vi "S8300E_Ping_Port1_WIH.vi"() -> ()   [LabVIEW 2011]
panel:
  out "PRELOG2":string
  out "PRELOG1":string
  out "KEYWORD2_AfterLogin":string
  out "log1":string
  out "Debug View":string
  out "VISA resource name out":refnum<visa-resource-name>
  out "Log":string
  out "IP list":cluster{"PORT3 IP":string, string}[](array[cluster])
  out "Msg":string
  out "Error Code List":string[](array[string])
  out "PORT3 IP":string
  out "PORT2 IP":string
  out "PORT1IP":string
  out "BEGIN TIME":u32
  out "進行狀況":string
  # "Error Code:NETPORT1\nError Code:NETPORT2\nError Code:NETPORT3"
  # "S8300E Ping port1 IP (接UART COM9)"
  # "2015-6-1"
  # "Step1:PING UUT PORT1 IP\nStep2:PING UUT PORT2 IP\nStep3:PING UUT PORT3 IP"
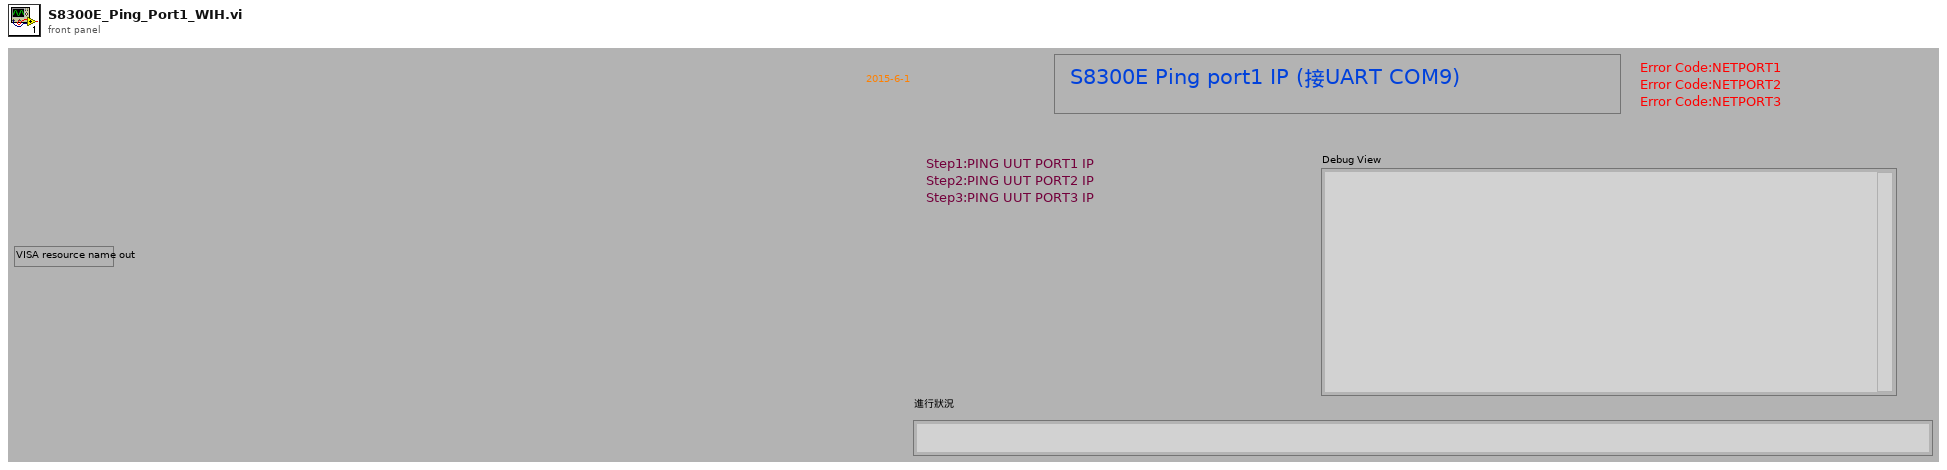
[diagram p1: front panel]
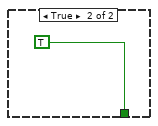
[diagram p6: hidden frame]
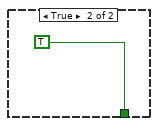
[diagram p9: hidden frame]
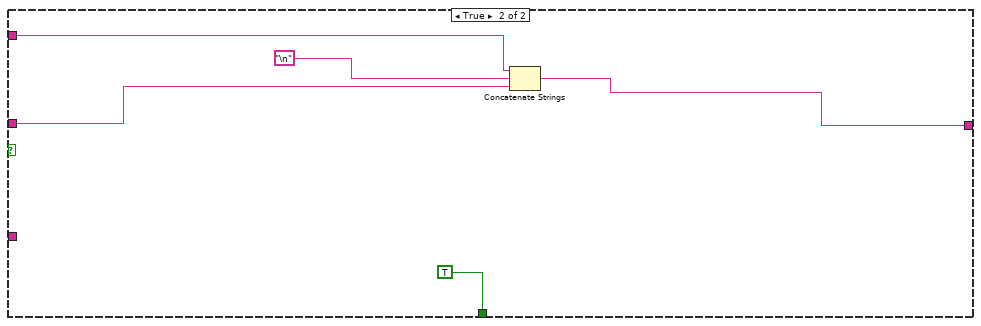
[diagram p11: hidden frame]
diagram:
  n1 = flat-sequence {
    tunnel: [w47] -> w3
    tunnel: [w46] -> w2
    tunnel: w3 -> [w53]
    tunnel: w2 -> [w52]
    tunnel: [w50] -> w1
    tunnel: w1 -> [w71]
    frame #0 {
      n2 = Tick Count (ms)() -> (millisecond timer value=→"BEGIN TIME":u32)
    }
    frame #1 {
      n3 = property on="進行狀況" class="Str"("Blinking"=TRUE) -> ()  [unwired: 2 in, 2 out]
      "進行狀況" <- "進入測試準備中...." ("進行狀況")
      "Debug View" <- ""
    }
    frame #2 {
      n4 = call "SUB_SearchFile_inFolder.vi"("Search Filename in Folder"="S8300E_sfcs_misc.txt") -> ("File Existing True/Flase"=w8:bool)  [unwired: 1 in]
      n5 = case shown="False" w8 {
        frame False {
          n6 = flat-sequence {
            frame #0 {
              n7 = call "Display Message to User"() -> ()  [unwired: 10 in, 2 out]
            }
            frame #1 {
              n8 = call "SUB_Writelog.vi"("Pass/Fail"="Fail:S8300E_Ping_Port1") -> ()  [unwired: 2 in]
            }
            frame #2 {
              n9 = Quit LabVIEW(quit? (T)=TRUE) -> ()
            }
          }
        }
        frame True {
        }
      }
    }
    frame #3 {
      w19 = "\r"
      n10 = call "SUB_ReadScript_File.vi"("Script FileName"="S8300E_sfcs_misc.txt" ("Search Filename in Folder")) -> ("text"=w16:string)  [unwired: 1 in, 2 out]
      n11 = call "SUB_FindSpecificString.vi"("Find this String"="TELNET_KEYWORD2_AFTERLOG_IN=", "String data"=w16) -> ("before \"; \" string"=→"KEYWORD2_AfterLogin":string, "Found"=w12:bool)  [unwired: 2 in]
      n12 = call "SUB_FindSpecificString.vi"("Find this String"="UUT_PORT2_IP=", "String data"=w16) -> ("before \"; \" string"=w22:string, "Found"=w26:bool)  [unwired: 2 in]
      "PORT2 IP" <- w22
      n13 = call "SUB_FindSpecificString.vi"("Find this String"="UUT_PORT3_IP=", "String data"=w16) -> ("before \"; \" string"=w21:string, "Found"=w24:bool)  [unwired: 2 in]
      "PORT3 IP" <- w21
      n14 = call "SUB_FindSpecificString.vi"("Find this String"="UUT_PORT1_IP=", "String data"=w16) -> ("before \"; \" string"=w23:string, "Found"=w27:bool)  [unwired: 2 in]
      "PORT1IP" <- w23
      n15 = And(x=w27, y=w26) -> (x .and. y?=w25:bool)
      n16 = Concatenate Strings("port IP不能設相同" ("Find this String"), w19, w23, w19, w22, w19, w21, w19) -> (→"Msg":string)
      n17 = And(x=w25, y=w24) -> (x .and. y?=w14:bool)
      n18 = And(x=w14, y=w12) -> (x .and. y?=w13:bool)
      n19 = case shown="False" w13 {
        frame False {
          n20 = flat-sequence {
            frame #0 {
              n21 = call "Display Message to User2"() -> ()  [unwired: 10 in, 2 out]
            }
            frame #1 {
              n22 = call "SUB_Writelog.vi"("Pass/Fail"="Fail:S8300E_Ping_Port1") -> ()  [unwired: 2 in]
            }
            frame #2 {
              n23 = Quit LabVIEW(quit? (T)=TRUE) -> ()
            }
          }
        }
        frame True {
        }
      }
    }
    frame #4 {
      n24 = local read "PORT1IP"() -> (w40:string)
      n25 = local read "PORT2 IP"() -> (w41:string)
      n26 = local read "PORT3 IP"() -> (w39:string)
      n27 = Equal?(x=w40, y=w41) -> (x = y?=w38:bool)
      n28 = Equal?(x=w41, y=w39) -> (x = y?=w37:bool)
      n29 = Equal?(x=w40, y=w39) -> (x = y?=w35:bool)
      n30 = Or(x=w38, y=w37) -> (x .or. y?=w36:bool)
      n31 = Or(x=w36, y=w35) -> (x .or. y?=w34:bool)
      n32 = case shown="True" w34 {
        frame False {
        }
        frame True {
          n33 = flat-sequence {
            frame #0 {
              n34 = local read "Msg"() -> (w42:string)
              n35 = call "Display Message to User3"("Message"=w42) -> ()  [unwired: 9 in, 2 out]
            }
            frame #1 {
              n36 = call "SUB_Writelog.vi"("Pass/Fail"="Fail:S8300E_Ping_Port1") -> ()  [unwired: 2 in]
            }
            frame #2 {
              n37 = Quit LabVIEW(quit? (T)=TRUE) -> ()
            }
          }
        }
      }
    }
    frame #5 {
      n38 = call "SUB_COM1_CLOSE.vi"("VISA resource name"=refnum<visa-resource-name> "COM9") -> ()  [unwired: 3 in]
    }
    frame #6 {
      n39 = call "SUB_COM9_INIT.vi"("baud rate"=u32 115200) -> ("VISA resource name out"=w47:refnum<visa-resource-name>)  [unwired: 1 in, 1 out]
      "VISA resource name out" <- w47
      n40 = Tick Count (ms)() -> (millisecond timer value=w46:u32)
    }
    frame #7 {
      n41 = while {
        tunnel: w53 -> [w68]
        tunnel: w52 -> [w65]
        shift-right: [w55] -> w49
        shift-left: "" -> [w61]
        tunnel: [w56] -> w50
        stop <- w60 stop-if-true
        n42 = Tick Count (ms)() -> (millisecond timer value=w66:u32)
        n43 = Subtract(x=w66, y=w65) -> (x-y=w64:u32)
        n44 = call "SUB_COM1Wrt.vi"("VISA resource name"=w68, "write buffer"="\r") -> ("duplicate VISA resource name"=w69:refnum<visa-resource-name>)  [unwired: 1 in, 1 out]
        n45 = Divide(x=w64, y=u32 1000) -> (x/y=w59:dbl)
        n46 = Greater Or Equal?(x=w59, y=2.0) -> (x >= y?=w57:bool)
        n47 = local read "KEYWORD2_AfterLogin"() -> (w54:string)
        n48 = call "SUB_ContinueCom1Read.vi"("Numeric"=50, "duplicate VISA resource name 2"=w69) -> ("String"=w62:string)  [unwired: 1 in, 2 out]
        n49 = Concatenate Strings(w61, w62) -> (w55:string)
        n50 = call "SUB_FindSpecificString.vi"("Find this String"=w54, "String data"=w55) -> ("Found"=w56:bool)  [unwired: 2 in, 1 out]
        n51 = local write "Debug View"(w55) -> ()
        n52 = Or(x=w56, y=w57) -> (x .or. y?=w60:bool)
      }
      "log1" <- w49
    }
    frame #8 {
      n53 = case shown="False" w71 {
        frame False {
          n54 = while {
            stop <- w81 stop-if-true
            n55 = local read "VISA resource name out"() -> (w73:refnum<visa-resource-name>)
            n56 = local read "KEYWORD2_AfterLogin"() -> (w75:string)
            n57 = Tick Count (ms)() -> (millisecond timer value=w78:u32)
            n58 = call "SUB_ContinueCom1Read.vi"("Numeric"=1200, "duplicate VISA resource name 2"=w73) -> ("duplicate VISA resource name"=w72:refnum<visa-resource-name>)  [unwired: 1 in, 2 out]
            n59 = call "SUB_WR_COM1_CbyCFindString_timeout.vi"("Begin time"=w78, "Find this String"=w75, "Timeout Seccond"=3.0, "cmd string"="\r", "duplicate VISA resource name 2"=w72) -> ("Output String"=w76:string, "Found String"=w77:bool)  [unwired: 2 out]
            n60 = case shown="False" w77 {
              tunnel: [w83 TRUE] -> w81
              tunnel: w76 -> [w82 _]
              frame False {
                n61 = call "SUB_YESNO.vi"("Debug View"=w82, "Status"="UART無正確反應!需有S8300E字串") -> ("yes/no"=w86:enum32{"No Selection", "Yes", "No", "None"})  [unwired: 1 in]
                n62 = Equal?(x=w86, y=enum32{"No Selection", "Yes", "No", "None"}."No") -> (x = y?=w84:bool)
                n63 = case shown="True" w84 {
                  tunnel: [_ w88] -> w83
                  frame False {
                  }
                  frame True {
                    n64 = flat-sequence {
                      tunnel: [w93] -> w88
                      frame #0 {
                        n65 = call "SUB_COM1_CLOSE.vi"("VISA resource name"=refnum<visa-resource-name> "COM9") -> ()  [unwired: 3 in]
                      }
                      frame #1 {
                        n66 = call "SUB_Writelog.vi"("Pass/Fail"="Fail:S8300E_Ping_Port1") -> ()  [unwired: 2 in]
                      }
                      frame #2 {
                        n67 = call "SUB_SFCS_SendResult.vi"("ErrorCode"="UART", "PASS_Fail (1/0)"=i8 0) -> ()  [unwired: 1 out]
                      }
                      frame #3 {
                        w93 = TRUE ("quit? (T)")
                        n68 = Quit LabVIEW(quit? (T)=w93) -> ()
                      }
                    }
                  }
                }
              }
              frame True {
              }
            }
          }
        }
        frame True {
        }
      }
    }
    frame #9 {
      n69 = while {
        stop <- w106 stop-if-true
        n70 = local read "VISA resource name out"() -> (w96:refnum<visa-resource-name>)
        n71 = call "SUB_ContinueCom1Read.vi"("Numeric"=1200, "duplicate VISA resource name 2"=w96) -> ("duplicate VISA resource name"=w95:refnum<visa-resource-name>)  [unwired: 1 in, 2 out]
        n72 = Concatenate Strings("./eth.sh -e  1", "\r") -> (w104:string)
        n73 = Tick Count (ms)() -> (millisecond timer value=w102:u32)
        n74 = call "SUB_WR_COM1_CbyCFindString_timeout.vi"("Begin time"=w102, "Find this String"="PASSED", "Timeout Seccond"=3.0, "cmd string"=w104, "duplicate VISA resource name 2"=w95) -> ("Output String"=w100:string, "Found String"=w101:bool)  [unwired: 2 out]
        n75 = case shown="False" w101 {
          tunnel: [w111 TRUE] -> w106
          tunnel: w100 -> [w109 _]
          frame False {
            w110 = "UART無正確反應!需有PASSED字串" ("Status")
            n76 = Concatenate Strings(w110, w109, "\n") -> (w107:string)
            n77 = call "SUB_YESNO.vi"("Debug View"=w109, "Status"=w110) -> ("yes/no"=w114:enum32{"No Selection", "Yes", "No", "None"})  [unwired: 1 in]
            n78 = Equal?(x=w114, y=enum32{"No Selection", "Yes", "No", "None"}."No") -> (x = y?=w112:bool)
            n79 = case shown="True" w112 {
              tunnel: [_ w116] -> w111
              tunnel: w107 -> [_ w115]
              frame False {
              }
              frame True {
                n80 = flat-sequence {
                  tunnel: w115 -> [w119]
                  tunnel: [w124] -> w116
                  frame #0 {
                    n81 = call "SUB_COM1_CLOSE.vi"("VISA resource name"=refnum<visa-resource-name> "COM9") -> ()  [unwired: 3 in]
                  }
                  frame #1 {
                    n82 = Concatenate Strings("Fail:S8300E_Ping_Port1" ("Pass/Fail"), "\n", w119) -> (w118:string)
                    n83 = call "SUB_Writelog.vi"("Pass/Fail"=w118) -> ()  [unwired: 2 in]
                  }
                  frame #2 {
                    n84 = call "SUB_SFCS_SendResult.vi"("ErrorCode"="UART", "PASS_Fail (1/0)"=i8 0) -> ()  [unwired: 1 out]
                  }
                  frame #3 {
                    w124 = TRUE ("quit? (T)")
                    n85 = Quit LabVIEW(quit? (T)=w124) -> ()
                  }
                }
              }
            }
          }
          frame True {
          }
        }
      }
    }
    frame #10 {
      n86 = Wait (ms)(milliseconds to wait=u32 1000) -> ()  [unwired: 1 out]
    }
    frame #11 {
      (unwired) "NETPORT3"
      (unwired) "NETPORT2"
      n87 = local read "PORT3 IP"() -> (w131:string)
      n88 = local read "PORT2 IP"() -> (w133:string)
      n89 = local read "PORT1IP"() -> (w137:string)
      n90 = Concatenate Strings("PING PORT2  ", w133) -> (w132:string)
      n91 = Concatenate Strings("PING PORT1  ", w137) -> (w136:string)
      n92 = Bundle("PORT1IP"=w137, w136) -> (w128:cluster{"PORT1IP":string, string})  [unwired: 1 in]
      n93 = Concatenate Strings("PING PORT3 ", w131) -> (w130:string)
      n94 = Bundle("PORT2 IP"=w133, w132) -> ()  [unwired: 1 in, 1 out]
      n95 = Bundle("PORT3 IP"=w131, w130) -> ()  [unwired: 1 in, 1 out]
      n96 = Build Array("NETPORT1") -> (→"Error Code List":string[])
      n97 = Build Array(w128) -> (→"IP list":cluster{"PORT1IP":string, string}[])
    }
    frame #12 {
      n98 = local read "IP list"() -> (w143:cluster{"PORT3 IP":string, string}[])
      n99 = Array Size(array=w143) -> (size(s)=w142:i32)
      n100 = for {
        N: w142 -> [_]
        shift-right: [w145] -> w140
        shift-left: "" -> [w144]
        i -> [w148]
        n101 = while {
          tunnel: w148 -> [w159]
          shift-right: [w152] -> w146
          shift-left: "" -> [w151]
          stop <- w155 stop-if-true
          n102 = local read "IP list"() -> (w161:cluster{"PORT3 IP":string, string}[])
          n103 = local read "Error Code List"() -> (w160:string[])
          n104 = Index Array(array=w161, index=w159) -> (element=w158:cluster{"PORT3 IP":string, string})
          n105 = Unbundle(w158) -> ("PORT3 IP"=w149:string, w157:string)
          n106 = Index Array(array=w160, index=w159) -> (element=w153:string)
          n107 = local write "進行狀況"(w157) -> ()
          n108 = call "SUB_Ping_IP_Status.vi"("IP Address"=w149) -> ("ok"=w156:bool, "standard output"=w154:string)
          n109 = case shown="False" w156 {
            tunnel: [_ TRUE] -> w155
            tunnel: w154 -> [w163 w188]
            tunnel: w153 -> [w166 _]
            tunnel: [w162 w187] -> w150
            tunnel: w149 -> [w165 w186]
            frame False {
              n110 = Concatenate Strings(w165, "\n", w163) -> (w162:string)
              n111 = call "SUB_YESNO.vi"("Debug View"=w163, "Status"="連線失敗!") -> ("yes/no"=w169:enum32{"No Selection", "Yes", "No", "None"})  [unwired: 1 in]
              n112 = Equal?(x=w169, y=enum32{"No Selection", "Yes", "No", "None"}."No") -> (x = y?=w167:bool)
              n113 = case shown="True" w167 {
                tunnel: w166 -> [_ w173]
                tunnel: w162 -> [_ w171]
                frame False {
                }
                frame True {
                  n114 = flat-sequence {
                    tunnel: [w174] -> w172
                    tunnel: w171 -> [w174]
                    tunnel: w172 -> [w176]
                    tunnel: w173 -> [w182]
                    frame #0 {
                      n115 = call "SUB_COM1_CLOSE.vi"("VISA resource name"=refnum<visa-resource-name> "COM9") -> ()  [unwired: 3 in]
                    }
                    frame #1 {
                      w177 = "\n"
                      n116 = local read "PRELOG2"() -> (w179:string)
                      n117 = local read "PRELOG1"() -> (w178:string)
                      n118 = Concatenate Strings("Fail:S8300E_Ping_Port1" ("Pass/Fail"), w177, w179, w177, w178, w177, w176) -> (w181:string)
                      n119 = call "SUB_Writelog.vi"("Pass/Fail"=w181) -> ()  [unwired: 2 in]
                    }
                    frame #2 {
                      n120 = call "SUB_SFCS_SendResult.vi"("ErrorCode"=w182, "PASS_Fail (1/0)"=i8 0) -> ()  [unwired: 1 out]
                    }
                    frame #3 {
                      n121 = Quit LabVIEW(quit? (T)=TRUE ("stop? (T)")) -> ()
                    }
                  }
                }
              }
            }
            frame True {
              n122 = Concatenate Strings(w186, "\n", w188) -> (w187:string)
            }
          }
          n123 = Concatenate Strings(w151, w150) -> (w152:string)
          "PRELOG1" <- w152
        }
        n124 = Concatenate Strings(w144, w146) -> (w145:string)
        "PRELOG2" <- w145
      }
      "Log" <- w140
    }
    frame #13 {
      w192 = "***Not Good ***" ("replace string (\"\")")
      n125 = local read "BEGIN TIME"() -> (w201:u32)
      n126 = Tick Count (ms)() -> (millisecond timer value=w200:u32)
      n127 = local read "Log"() -> (w197:string)
      n128 = call "SUB_CAL_TESTTIME.vi"("Test Item name"="S8300E_Ping_Port1", "Stop tick time"=w200, "Start tick time"=w201) -> ("Test Time output"=w196:string)  [unwired: 2 in]
      n129 = Concatenate Strings("Pass:S8300E_Ping_Port1", "\n", w197, w196) -> (w191:string)
      n130 = call "SUB_SEARCH_REPLACE_STR.vi"("replace string (\"\")"=w192, "search string"="FAILED", "input string"=w191) -> ("result string"=w194:string)  [unwired: 2 in]
      n131 = call "SUB_SEARCH_REPLACE_STR.vi"("replace string (\"\")"=w192, "search string"="FAIL", "input string"=w194) -> ("result string"=w190:string)  [unwired: 2 in]
      n132 = call "SUB_Writelog.vi"("Pass/Fail"=w190) -> ()  [unwired: 2 in]
    }
    frame #14 {
      n133 = call "SUB_COM1_CLOSE.vi"("VISA resource name"=refnum<visa-resource-name> "COM9") -> ()  [unwired: 3 in]
    }
    frame #15 {
      n134 = Request Deallocation(TRUE ("flag")) -> ()
    }
    frame #16 {
      n135 = Quit LabVIEW(quit? (T)=TRUE ("stop? (T)")) -> ()
    }
  }
